vi "Display Panel VI.vi"(11 "Display Panel Non-Actor Class.lvlib:Display Panel Non-Actor Class.lvclass":refnum<class "Display Panel Non-Actor Class.lvclass">) -> (3 "Display Panel Non-Actor Class out":refnum<class "Display Panel Non-Actor Class.lvclass">)   [LabVIEW 2013]
uses:
  Controls/Numeric Indicator.ctl
  Display panel Non-Actor Class/Display Panel Non-Actor Class.lvclass
panel:
  out "error out":errorcluster
  in  "error in (no error)":errorcluster
  out "card #":dbl
  out "iteration #":i32
  out "Display Input":T1[](array[typedef])
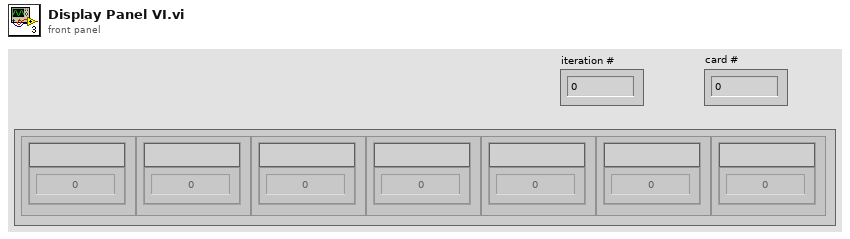
[diagram p1: front panel]
types:
  T1 = typedef "Numeric Indicator.ctl" = cluster{"Numeric Indicator 2":dbl, "String":string}
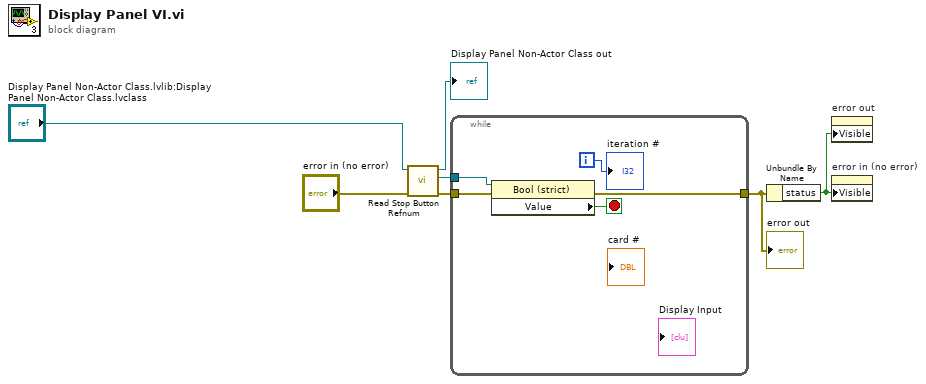
[diagram p0: block diagram]
diagram:
  n1 = call-dynamic "Read Stop Button Refnum.vi"("error in (no error)"="error in (no error)", "Display Panel Non-Actor Class in"="Display Panel Non-Actor Class.lvlib:Display Panel Non-Actor Class.lvclass") -> ("error out"=w3:errorcluster, "Stop Button Refnum"=w6:refnum<vi>, "Display Panel Non-Actor Class out"=→"Display Panel Non-Actor Class out":refnum<class "Display Panel Non-Actor Class.lvclass">)  [unwired: 7 in]
  n2 = while {
    tunnel: w6 -> [w11]
    tunnel: w3 -> [w9]
    tunnel: [w8] -> w2
    i -> [w12]
    stop <- w10 stop-if-true
    n3 = property class="Bool (strict)"(reference=w11, error in=w9) -> (error out=w8:errorcluster, "Value"=w10:bool)  [unwired: 1 out]
    "iteration #" <- w12
  }
  "error out" <- w2
  n4 = Unbundle By Name(w2) -> ("status"=w1:bool)
  n5 = property on="error out" class="Clust (strict)"("Visible"=w1) -> ()  [unwired: 2 in, 2 out]
  n6 = property on="error in (no error)" class="Clust (strict)"("Visible"=w1) -> ()  [unwired: 2 in, 2 out]
